vi "Page_Source_New_Configurable_VI.vi"(8 "error in (no error)":errorcluster, 11 "AB_Build in":refnum<class "AB_Build.lvclass">) -> (0 "error out":errorcluster, 2 "AB_Source_VI out":refnum<class "AB_Source_VI.lvclass">, 3 "AB_Build out":refnum<class "AB_Build.lvclass">)   [LabVIEW 2020, in "AB_Build.lvclass"]
uses:
  <vilib>/AppBuilder/AB_Classes/Build/AB_Build.lvclass
  <vilib>/AppBuilder/AB_Classes/Source/VI/AB_Source_VI.lvclass
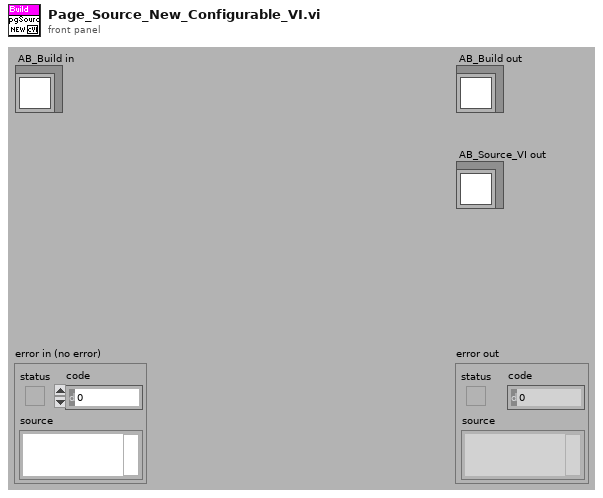
[diagram p1: front panel]
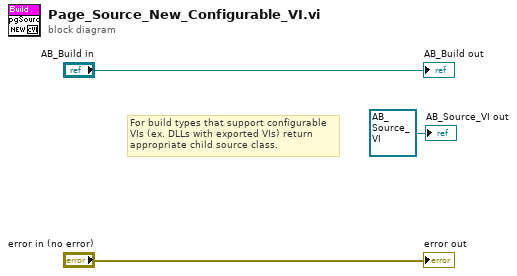
[diagram p0: block diagram]
diagram:
  # "For build types that support configurable VIs (ex. DLLs with exported VIs) return appropriate child source class."
  "error out" <- "error in (no error)"
  "AB_Build out" <- "AB_Build in"
  "AB_Source_VI out" <- refnum<class "AB_Source_VI.lvclass"> refnum ("AB_Source_VI out")
